vi "process.vi"(8 "error in (no error)":errorcluster, 9 "Calling VI Reference i":refnum<vi>, 10 "Node Refnum":refnum<vi>, 11 "MultiFrameStructure in":refnum<class "MultiFrameStructure.lvclass">) -> (0 "error out":errorcluster, 3 "MultiFrameStructure out":refnum<class "MultiFrameStructure.lvclass">)   [LabVIEW 2016, in "MultiFrameStructure.lvclass"]
uses:
  MultiFrameStructure.lvclass
  C:/LSST_TS/SystemSW/ct_tools/Node/Node.lvclass
  Dependency/Dependency.lvclass
  Node/Node.lvclass/Node.ctl
  Dependency/Dependency.lvclass/Dependency.ctl
  Node/Node.lvclass
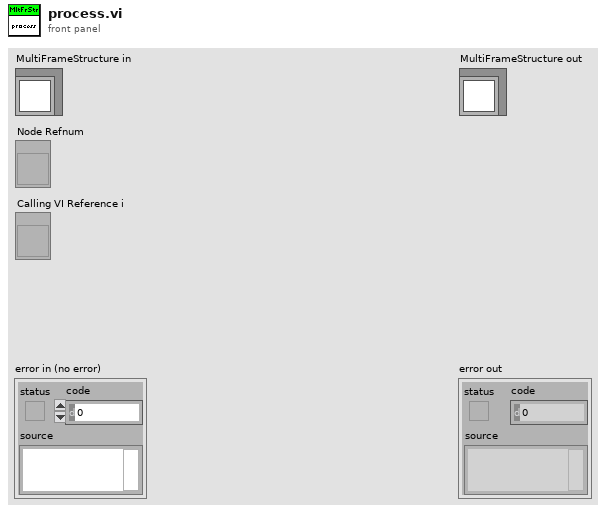
[diagram p1: front panel]
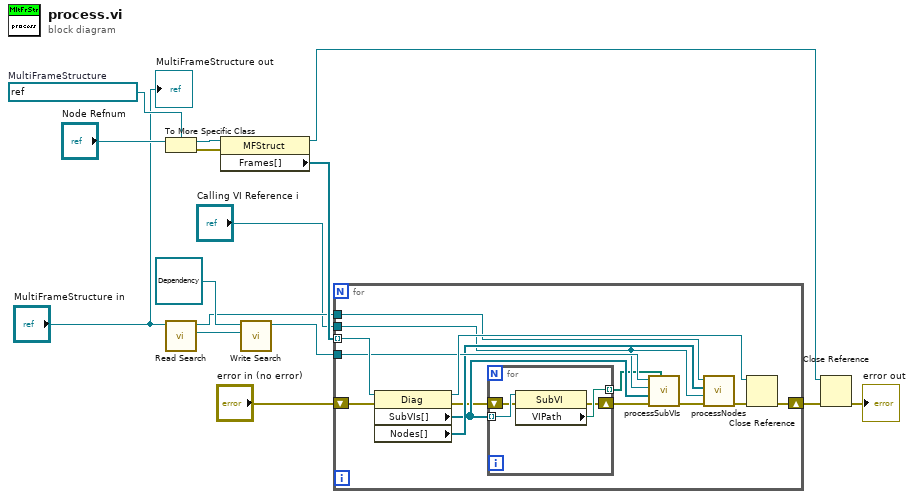
[diagram p0: block diagram]
diagram:
  w12 = refnum<vi> refnum  # MultiFrameStructure
  n1 = To More Specific Class(target class=w12, reference="Node Refnum") -> (specific class reference=w15:refnum<vi>, error out=w14:errorcluster)  [unwired: 1 in]
  n2 = call "Read Search.vi"("Node in"="MultiFrameStructure in") -> ("Search"=w7:refnum<class "Search.lvclass">, "Node out"=w6:refnum<class "MultiFrameStructure.lvclass">)  [unwired: 9 in]
  n3 = property class="MFStruct"(reference=w15, error in=w14) -> (reference out=w10:refnum<vi>, "Frames[]"=w13:refnum<vi>[])  [unwired: 1 out]
  n4 = call "Write Search.vi"("Search"=w7, "Dependency in"=refnum<class "Dependency.lvclass"> refnum ("Dependency.lvclass")) -> ("Dependency out"=w8:refnum<class "Dependency.lvclass">)  [unwired: 9 in]
  n5 = for {
    tunnel: w13 -> [w29] mode=indexing
    tunnel: "Calling VI Reference i" -> [w20]
    shift-right: [w26] -> w11
    shift-left: "error in (no error)" -> [w28]
    tunnel: w8 -> [w25]
    tunnel: w6 -> [w24]
    n6 = property class="Diag"(reference=w29, error in=w28) -> (reference out=w27:refnum<vi>, error out=w17:errorcluster, "SubVIs[]"=w19:refnum<vi>[], "Nodes[]"=w23:refnum<vi>[])
    n7 = for {
      tunnel: w19 -> [w33] mode=indexing
      tunnel: [w32] -> w18 mode=indexing
      shift-right: [w31] -> w16
      shift-left: w17 -> [w30]
      n8 = property class="SubVI"(reference=w33, error in=w30) -> (error out=w31:errorcluster, "VIPath"=w32:path)  [unwired: 1 out]
    }
    n9 = call "processSubVIs.vi"("VIDependencyPaths"=w18, "error in (no error)"=w16, "SubVIs[]"=w19, "Calling VI Reference i"=w20, "Dependency in"=w25) -> ("error out"=w22:errorcluster)  [unwired: 4 in, 2 out]
    n10 = call "processNodes.vi"("error in (no error)"=w22, "Calling VI Reference i"=w20, "Nodes[]"=w23, "Node in"=w24) -> ("error out"=w21:errorcluster)  [unwired: 6 in, 1 out]
    n11 = Close Reference(reference=w27, error in (no error)=w21) -> (error out=w26:errorcluster)
  }
  n12 = Close Reference(reference=w10, error in (no error)=w11) -> (error out=→"error out":errorcluster)
  "MultiFrameStructure out" <- "MultiFrameStructure in"
